vi "libssh2_info.vi"() -> ()   [LabVIEW 2013]
doc: "Illustrates how to get information about your version of libssh2."
uses:
  libssh2/libssh2_init_custom.vi
  libssh2/libssh2_init_default.vi
  libssh2/libssh2.lvlib
panel:
  out "error out":errorcluster
  out "crypto engine":T1(ring)
  out "version":string
  in  "Path to libssh2 (\"\" = default)":path
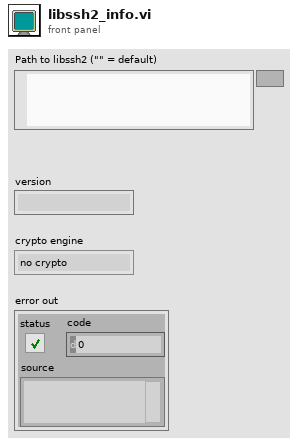
[diagram p1: front panel]
types:
  T1 = enum16{"no crypto", "OpenSSL", "gcrypt", "mbedTLS", "WinCNG", "OS400qc3"}
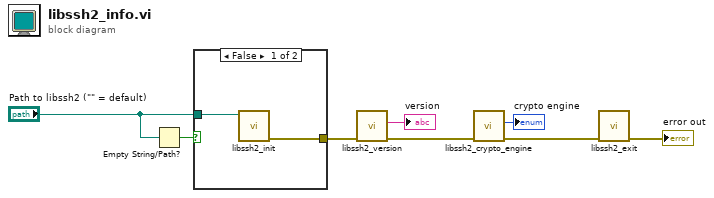
[diagram p0: block diagram]
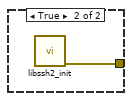
[diagram p2: hidden frame]
diagram:
  n1 = Empty String/Path?(string/path="Path to libssh2 (\"\" = default)") -> (empty?=w8:bool)
  n2 = case shown="False" w8 {
    tunnel: "Path to libssh2 (\"\" = default)" -> [w10 _]
    tunnel: [w9 w11] -> w6
    frame False {
      n3 = call-poly "libssh2_init.vi"("path (use built-in)"=w10) -> ("error out"=w9:errorcluster)  [unwired: 10 in]
    }
    frame True {
      n4 = call-poly "libssh2_init.vi"() -> ("error out"=w11:errorcluster)  [unwired: 11 in]
    }
  }
  n5 = call "libssh2_version.vi"("error in (no error)"=w6) -> ("error out"=w5:errorcluster, "version"=→"version":string)  [unwired: 9 in]
  n6 = call "libssh2_crypto_engine.vi"("error in (no error)"=w5) -> ("error out"=w3:errorcluster, "crypto engine"=→"crypto engine":T1)  [unwired: 9 in]
  n7 = call "libssh2_exit.vi"("error in (no error)"=w3) -> ("error out"=→"error out":errorcluster)  [unwired: 10 in]
